vi "GetIniInfo.vi"(8 "error in (no error)":errorcluster, 10 "Base Path":path, 11 "Path to Plugin INI":path) -> (0 "error out":errorcluster, 2 "DefaultINIParams":T1={"Handle"="", "eFunction"=0, "dRange"=0.0, "dResolution"=0.0, "eTriggerSource"=0, "dTriggerDelay"=0.0, "iMaxTimeMilliseconds"=0, "eMeasCompleteDest"=0, "iTriggerCount"=0, "iSampleCount"=0, "eSampleClock"=0, "dSampleInterval"=0.0, "iMaxTimeMillisecondsMultiPoint"=0, "iArraySize"=0, "dMinFreq"=0.0, "dMaxFreq"=0.0, "dFrequencyVoltageRange"=0.0, "eEdge"=10280, "sSource"="", "eEdgeSample"=10280, "sSourceSample"="", "eSampleMode"=10178} {"eSampleMode" items=["Finite Samples"=10178, "Continuous Samples"=10123, "Hardware Timed Single Point"=12522]; "eEdgeSample" items=["Rising"=10280, "Falling"=10171]; "eEdge" items=["Rising"=10280, "Falling"=10171]; "eSampleClock" items=["NULL"=0, "Immediate"=1, "External"=2, "Software Trigger"=3, "Interval"=10]; "eMeasCompleteDest" items=["None"=0, "External"=2]; "eTriggerSource" items=["NULL", "Immediate", "External", "Software Trigger"]; "eFunction" items=["NULL"=0, "DC Volts"=1, "AC Volts"=2, "DC Current"=3, "AC Current"=4, "Frequency"=104, "AC Coupled Direct Sampling"=1005]}, 3 "Path to Class":path)   [LabVIEW 2014]
uses:
  SamplerPluginsBase.lvclass
  <userlib>/NIST/BaseClasses/Object_class/BaseObject.lvclass
  TypeDefs/DefaultINIParams.ctl
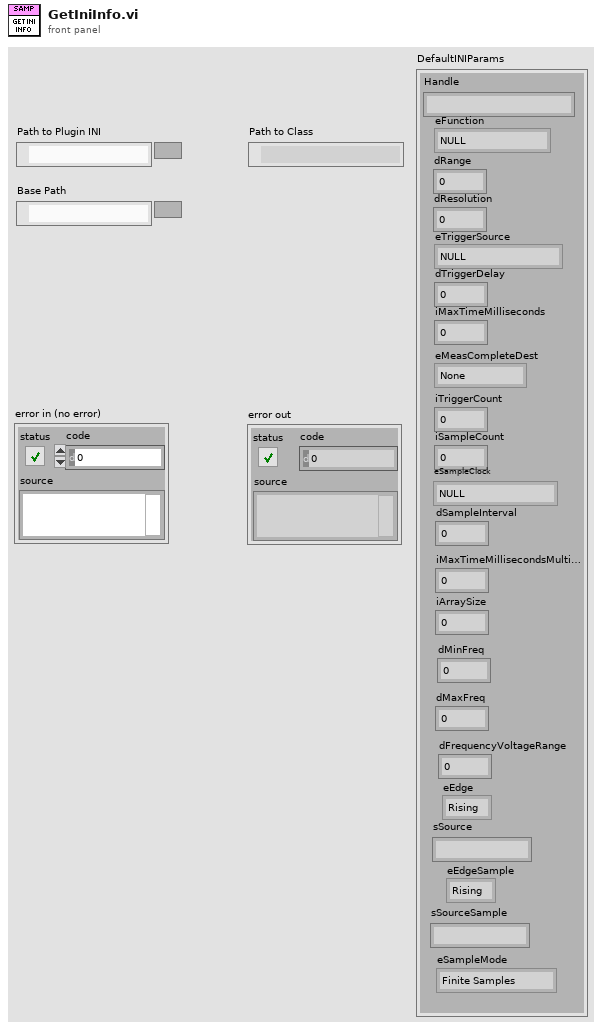
[diagram p1: front panel]
types:
  T1 = typedef "SamplerPlugins.lvlib/SamplerPluginsBase.lvclass/DefaultINIParams.ctl" = cluster{"Handle":string, "eFunction":u16, "dRange":dbl, "dResolution":dbl, "eTriggerSource":u16, "dTriggerDelay":dbl, "iMaxTimeMilliseconds":i32, "eMeasCompleteDest":u16, "iTriggerCount":i32, "iSampleCount":i32, "eSampleClock":u16, "dSampleInterval":dbl, "iMaxTimeMillisecondsMultiPoint":i32, "iArraySize":i32, "dMinFreq":dbl, "dMaxFreq":dbl, "dFrequencyVoltageRange":dbl, "eEdge":u16, "sSource":string, "eEdgeSample":u16, "sSourceSample":string, "eSampleMode":i32}
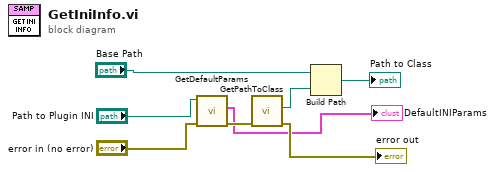
[diagram p0: block diagram]
diagram:
  n1 = call "GetDefaultParams.vi"("error in (no error)"="error in (no error)", "config file path"="Path to Plugin INI") -> ("error out"=w3:errorcluster, "DefaultINIParams"=→"DefaultINIParams":T1)  [unwired: 8 in]
  n2 = call <userlib>:"GetPathToClass.vi"("error in (no error)"=w3) -> ("error IO"=→"error out":errorcluster, "PathToClass"=w7:path)  [unwired: 9 in]
  n3 = Build Path(base path="Base Path", name or relative path=w7) -> (appended path=→"Path to Class":path)
